vi "FA_Close.vi"(8 "Error In":errorcluster, 11 "FA_LS Ref":T1) -> (0 "Error Out":errorcluster)   [LabVIEW 2013, in "FA_LocalStore.lvlib"]
doc: "Closes all XML references and the eTag INI file reference. Does not obey standard error in behavior. This is done to ensure we do not leak references when error do occur."
uses:
  FA_LocalStore.lvlib
  FA_LSRef.ctl
  <vilib>/Utility/config.llb/Config Data RefNum.ctl
  <vilib>/Utility/config.llb/NI_LVConfig.lvlib
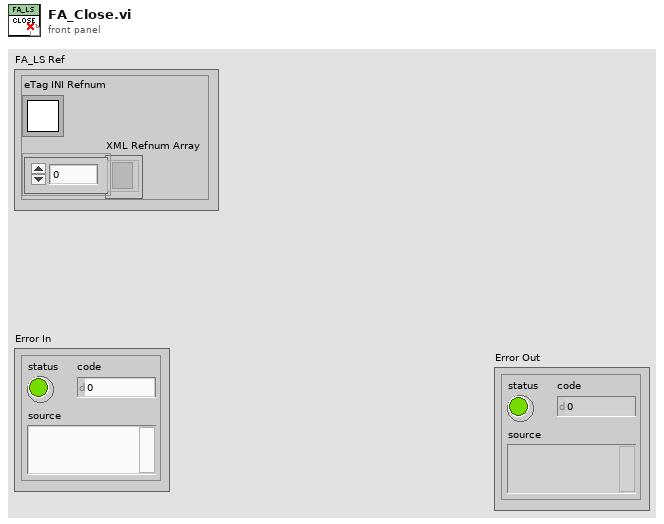
[diagram p1: front panel]
types:
  T1 = typedef "FA_LocalStore.lvlib/FA_LSRef.ctl" = cluster{"eTag INI Refnum":T2, "XML Refnum Array":refnum<file>[]}
  T2 = typedef "NI_LVConfig.lvlib/Config Data RefNum.ctl" = refnum<k1>
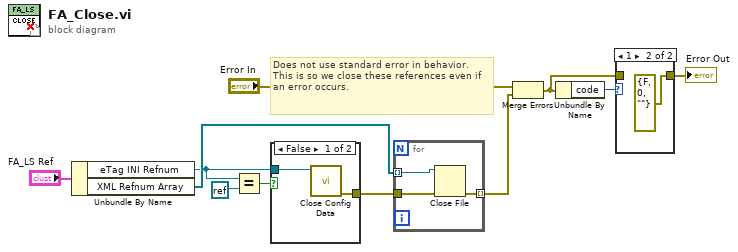
[diagram p0: block diagram]
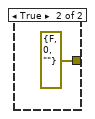
[diagram p3: hidden frame]
diagram:
  # "Does not use standard error in behavior.  This is so we close these references even if an error occurs."
  n1 = Unbundle By Name("FA_LS Ref") -> ("eTag INI Refnum"=w4:T2, "XML Refnum Array"=w7:refnum<file>[])
  n2 = Equal?(x=w4, y=refnum<k0> refnum) -> (x = y?=w5:bool)
  n3 = case shown="False" w5 {
    tunnel: [w13 errorcluster {"status"=FALSE, "code"=0, "source"=""} ("error out")] -> w10
    tunnel: w4 -> [w12 _]
    frame False {
      n4 = call <vilib>:"Close Config Data.vi"("refnum"=w12) -> ("error out"=w13:errorcluster)  [unwired: 9 in, 1 out]
    }
    frame True {
    }
  }
  n5 = for {
    tunnel: w10 -> [w17]
    tunnel: [w16] -> w8 mode=indexing
    tunnel: w7 -> [w15] mode=indexing
    n6 = Close File(refnum=w15, error in=w17) -> (error out=w16:errorcluster)  [unwired: 1 out]
  }
  n7 = Merge Errors("Error In", w8) -> (w1:errorcluster)
  n8 = Unbundle By Name(w1) -> ("code"=w3:i32)
  n9 = case shown="1" w3 {
    tunnel: [w18 errorcluster {"status"=FALSE, "code"=0, "source"=""} ("error out")] -> w2
    tunnel: w1 -> [w18 _]
    frame 0, Default {
    }
    frame 1 {
    }
  }
  "Error Out" <- w2
